vi "Init HTTP.vi"(8 "error in (no error)":errorcluster, 11 "Hardware Info Module in":refnum<class "Hardware Info Module.lvclass">) -> (0 "error out":errorcluster, 3 "Hardware Info Module out":refnum<class "Hardware Info Module.lvclass">)   [LabVIEW 2023, in "Volatus.lvlib" / "Hardware Info Module.lvclass"]
uses:
  Hardware Info Module.lvclass
  Module/Module.lvclass/Module.ctl
  VolatusAPI/VolatusAPI.lvclass/VolatusAPI.ctl
  lv-http-server/HTTP Server/Server/Register Handler.vi
  HardwareHTTPController/HardwareHTTPController.lvclass
  lv-vecto/Vecto/Vecto/Get HTTP.vi
  lv-http-server/HTTP Server/Server/Add Connection Handler.vi
  lv-http-server/HTTP Server/Server/Add Request Handler.vi
  lv-http-server/HTTP Server/Server/Add Route Handler.vi
  lv-http-server/HTTP Server/Server/Add Controller Handler.vi
  lv-http-server/HTTP Server/Server/Add Controller.vi
  lv-http-server/HTTP Server/Server/Add Response Handler.vi
  lv-http-server/HTTP Server/Server/Add Complete Handler.vi
  lv-http-server/HTTP Server/Server/Add Exception Handler.vi
  lv-http-server/HTTP Server/Connection Handler/Connection Handler.lvclass
  lv-http-server/HTTP Server/Request Handler/Request Handler.lvclass
  lv-http-server/HTTP Server/Route Handler/Route Handler.lvclass
  lv-http-server/HTTP Server/Controller Handler/Controller Handler.lvclass
  lv-http-server/HTTP Server/Controller/Controller.lvclass
  lv-http-server/HTTP Server/Response Handler/Response Handler.lvclass
  lv-http-server/HTTP Server/Complete Handler/Complete Handler.lvclass
  lv-http-server/HTTP Server/Exception Handler/Exception Handler.lvclass
  lv-http-server/HTTP Server/Handler/Handler.lvclass
  Hardware Info Module.lvclass/Hardware Info Module.ctl
  Module/Module.lvclass
  VolatusAPI/VolatusAPI.lvclass
  C:/dev/volatus/mts-volatus-super/libs/lv-volatus/Volatus/Module/Module.lvclass
  C:/dev/volatus/mts-volatus-super/libs/lv-volatus/Volatus/Hardware Info Module/Hardware Info Module.lvclass
  Nav Route/Nav Route.lvclass
  C:/dev/volatus/mts-volatus-super/libs/lv-http-server/HTTP Server/Controller/Controller.lvclass
  C:/dev/volatus/mts-volatus-super/libs/lv-http-server/HTTP Server/Handler/Handler.lvclass
  C:/dev/volatus/mts-volatus-super/libs/lv-volatus/Volatus/HardwareHTTPController/HardwareHTTPController.lvclass
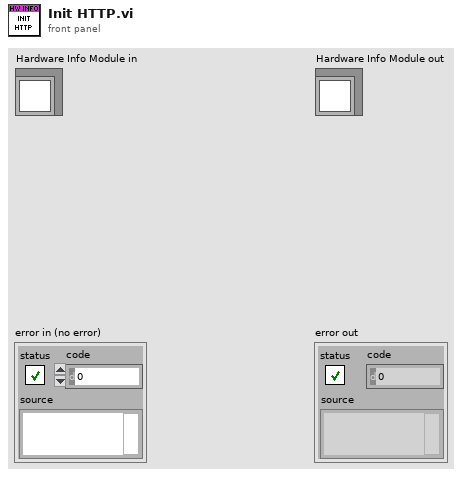
[diagram p1: front panel]
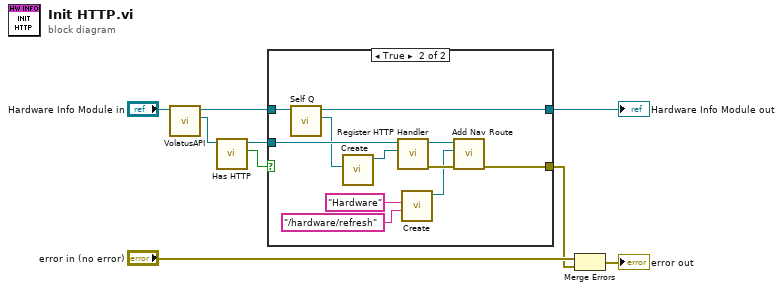
[diagram p0: block diagram]
diagram:
  n1 = call "VolatusAPI.vi"("Module in"="Hardware Info Module in") -> ("VolatusAPI"=w7:refnum<class "VolatusAPI.lvclass">, "Module out"=w5:refnum<class "Hardware Info Module.lvclass">)  [unwired: 9 in]
  n2 = call "Has HTTP.vi"("VolatusAPI in"=w7) -> ("Has HTTP"=w4:bool, "VolatusAPI out"=w3:refnum<class "VolatusAPI.lvclass">)  [unwired: 9 in]
  n3 = case shown="True" w4 {
    tunnel: [w10 w21] -> w8
    tunnel: w5 -> [w10 w20]
    tunnel: w3 -> [_ w19]
    tunnel: [_ w11] -> w1
    frame False {
    }
    frame True {
      n4 = call "Self Q.vi"("Module in"=w20) -> ("Self Q"=w18:refnum<class "MessageQ.lvclass">, "Module out"=w21:refnum<class "Hardware Info Module.lvclass">)  [unwired: 9 in]
      n5 = call "Create.vi"("MsgQ"=w18) -> ("HardwareHTTPController out"=w17:refnum<class "HardwareHTTPController.lvclass">)  [unwired: 9 in, 1 out]
      n6 = call "Register HTTP Handler.vi"("Handler"=w17, "VolatusAPI in"=w19) -> ("error out"=w16:errorcluster, "VolatusAPI out"=w15:refnum<class "VolatusAPI.lvclass">)  [unwired: 8 in]
      n7 = call "Create.vi"("Path"="/hardware/refresh" ("Label"), "Label"="Hardware") -> ("Nav Route out"=w12:refnum<class "Nav Route.lvclass">)  [unwired: 8 in, 1 out]
      n8 = call "Add Nav Route.vi"("error in (no error)"=w16, "Nav Route"=w12, "VolatusAPI in"=w15) -> ("error out"=w11:errorcluster)  [unwired: 7 in, 1 out]
    }
  }
  "Hardware Info Module out" <- w8
  n9 = Merge Errors("error in (no error)", w1) -> (→"error out":errorcluster)
